vi "Initialize CAN FD.vi"(8 "error in":errorcluster, 10 "BitrateFD":string="f_clock=80000000,nom_brp=2,nom_tseg1=63,nom_tseg2=16,nom_sjw=16,data_brp=2,data_tseg1=15,data_tseg2=4,data_sjw=4", 11 "Channel":u16) -> (0 "error out":errorcluster, 3 "Channel out":u16)   [LabVIEW 2025, in "PCAN API.lvlib"]
uses:
  PCAN API.lvlib
  PCAN2023/PCAN2023.lvlib
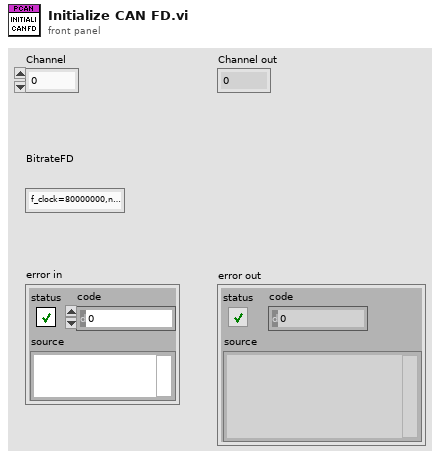
[diagram p1: front panel]
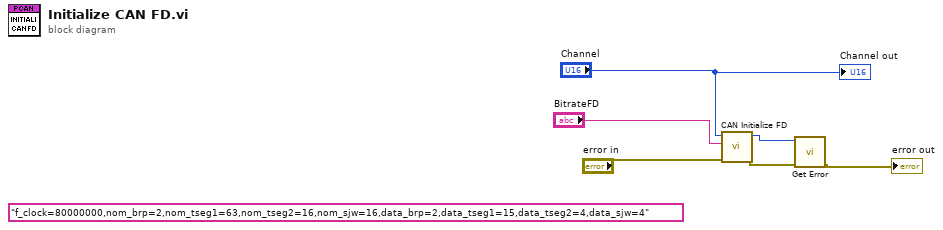
[diagram p0: block diagram]
diagram:
  (unwired) "f_clock=80000000,nom_brp=2,nom_tseg1=63,nom_tseg2=16,nom_sjw=16,data_brp=2,data_tseg1=15,data_tseg2=4,data_sjw=4" ("BitrateFD")
  n1 = call "CAN Initialize FD.vi"("error in (no error)"="error in", "BitrateFD"="BitrateFD", "Channel"="Channel") -> ("error out"=w6:errorcluster, "function return"=w5:u32)  [unwired: 6 in, 1 out]
  n2 = call "Get Error.vi"("error in (no error)"=w6, "function return"=w5) -> ("error out"=→"error out":errorcluster)  [unwired: 9 in]
  "Channel out" <- "Channel"
